vi "FF_JK.vi"(2 "K":bool, 3 "Clock":bool, 4 "J":bool) -> (0 "Q!":bool, 1 "Q":bool)   [LabVIEW 2018]
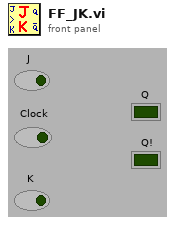
[diagram p1: front panel]
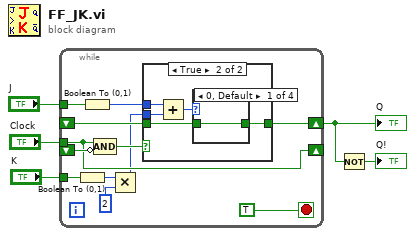
[diagram p0: block diagram]
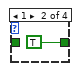
[diagram p3: hidden frame]
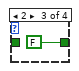
[diagram p4: hidden frame]
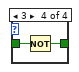
[diagram p5: hidden frame]
diagram:
  n1 = while {
    tunnel: "J" -> [w14]
    shift-right: [w16] -> _
    shift-left: _ -> [w17]
    shift-right: [w10] -> w1
    shift-left: _ -> [w11]
    tunnel: "Clock" -> [w16]
    tunnel: "K" -> [w13]
    stop <- TRUE stop-if-true
    n2 = Boolean To (0,1)(Boolean=w13) -> (0, 1=w8:i16)
    n3 = Boolean To (0,1)(Boolean=w14) -> (0, 1=w9:i16)
    n4 = Compound Arithmetic op=AND(w16, invert w17) -> (w12:bool)
    n5 = Multiply(x=w8, y=i16 2) -> (x*y=w6:i16)
    n6 = case shown="True" w12 {
      tunnel: w11 -> [w18 w20]
      tunnel: [w18 w21] -> w10
      tunnel: w9 -> [_ w23]
      tunnel: w6 -> [_ w19]
      frame False {
      }
      frame True {
        n7 = Add(x=w23, y=w19) -> (x+y=w22:i16)
        n8 = case shown="0, Default" w22 {
          tunnel: [w24 TRUE FALSE w28] -> w21
          tunnel: w20 -> [w24 _ _ w27]
          frame 0, Default {
          }
          frame 1 {
          }
          frame 2 {
          }
          frame 3 {
            n9 = Not(x=w27) -> (.not. x?=w28:bool)
          }
        }
      }
    }
  }
  "Q" <- w1
  n10 = Not(x=w1) -> (.not. x?=→"Q!":bool)
